vi "Shutdown.vi"(8 "error in":errorcluster, 11 "Launcher in":refnum<class "Launcher.lvclass">) -> (0 "error out":errorcluster, 3 "Launcher out":refnum<class "Launcher.lvclass">)   [LabVIEW 2023, in "Launcher.lvlib" / "Launcher.lvclass"]
uses:
  Library/Launcher.lvclass
  Library/Launcher.lvclass/Launcher.ctl
  builds/Base Software/Base Software.lvlibp/Base Software Messages/Respond to Menu Event Msg/Respond to Menu Event Msg.lvclass
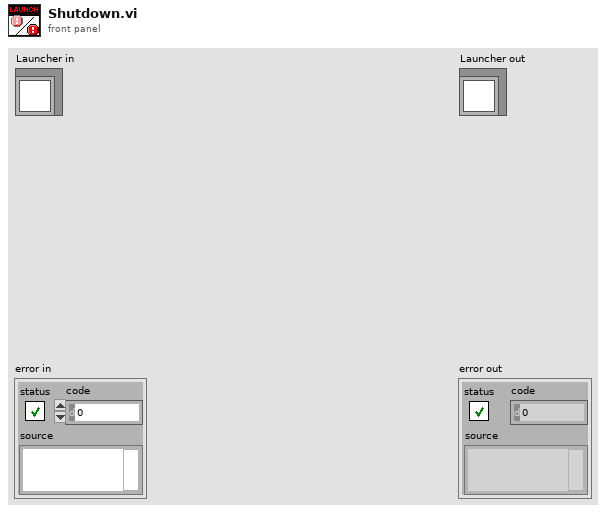
[diagram p1: front panel]
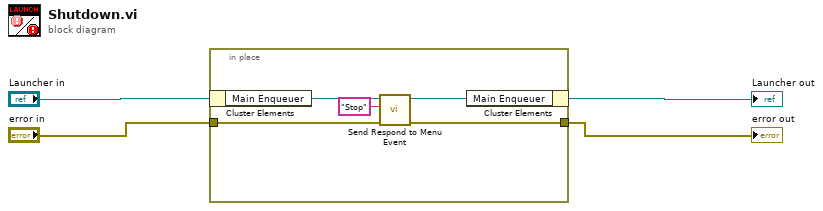
[diagram p0: block diagram]
diagram:
  n1 = in-place {
    in-place-border: [w6] -> w2
    in-place-border: "error in" -> [w5]
    n2 = in-place-cluster #1("Launcher in") -> ("Main Enqueuer"=w9:refnum<class "Message Enqueuer.lvclass">)
    n3 = call "Send Respond to Menu Event.vi"("error in (no error)"=w5, "Selection"="Stop", "Message Enqueuer"=w9) -> ("error out"=w6:errorcluster, "Message Enqueuer out"=w8:refnum<class "Message Enqueuer.lvclass">)  [unwired: 7 in]
    n4 = in-place-cluster #1("Main Enqueuer"=w8) -> (→"Launcher out":refnum<class "Launcher.lvclass">)
  }
  "error out" <- w2
